vi "Get Ctrl Value.vi"(8 "error in (no error)":errorcluster, 11 "Ctrl Refnum Column in":refnum<class "Ctrl Refnum Column.lvclass">) -> (0 "error out":errorcluster, 2 "Ctrl Value":variant, 3 "Ctrl Refnum Column out":refnum<class "Ctrl Refnum Column.lvclass">)   [LabVIEW 2020, in "Basic Fields.lvlib" / "Ctrl Refnum Column.lvclass"]
uses:
  Ctrl Refnum Column.lvclass
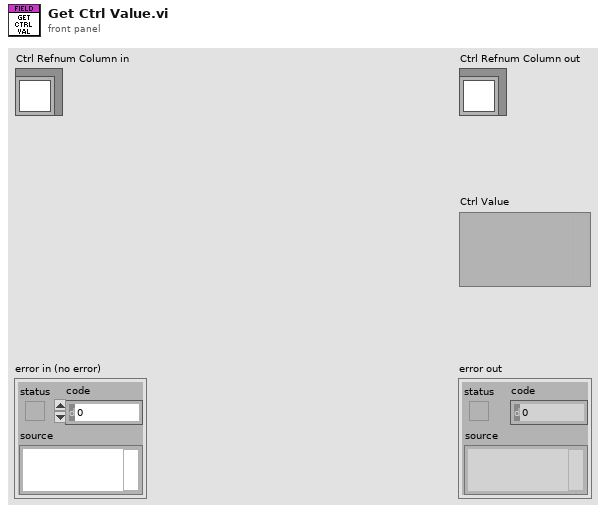
[diagram p1: front panel]
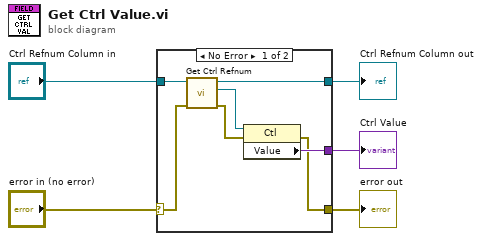
[diagram p0: block diagram]
diagram:
  n1 = case shown="No Error" "error in (no error)" {
    selector: "error in (no error)" -> [w8 w14]
    tunnel: [w6 w14] -> w4
    tunnel: [w11 w13] -> w2
    tunnel: "Ctrl Refnum Column in" -> [w12 w13]
    tunnel: [w9 _] -> w1
    frame No Error {
      n2 = call-dynamic "Get Ctrl Refnum.vi"("error in (no error)"=w8, "Ctrl Refnum Column in"=w12) -> ("error out"=w7:errorcluster, "Ctl Refnum"=w10:refnum<vi>, "Ctrl Refnum Column out"=w11:refnum<class "Ctrl Refnum Column.lvclass">)  [unwired: 7 in]
      n3 = property class="Ctl"(reference=w10, error in=w7) -> (error out=w6:errorcluster, "Value"=w9:variant)  [unwired: 1 out]
    }
    frame Error {
    }
  }
  "error out" <- w4
  "Ctrl Refnum Column out" <- w2
  "Ctrl Value" <- w1
